vi "CMI LiB Bias Open.vi"(8 "error in":errorcluster, 10 "reset (false)":bool, 11 "VISA in":refnum<visa-resource-name>) -> (0 "error out":errorcluster, 2 "idn string":string, 3 "VISA out":refnum<visa-resource-name>)   [LabVIEW 2020]
uses:
  <vilib>/Utility/error.llb/Error Cluster From Error Code.vi
  <vilib>/ErrorRing/Error Ring.xnode
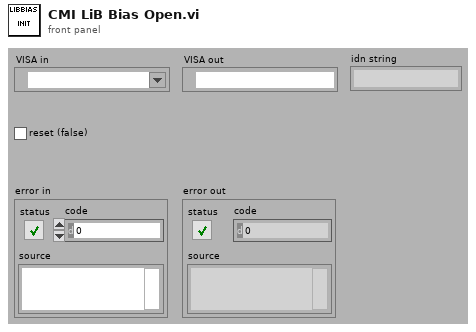
[diagram p1: front panel]
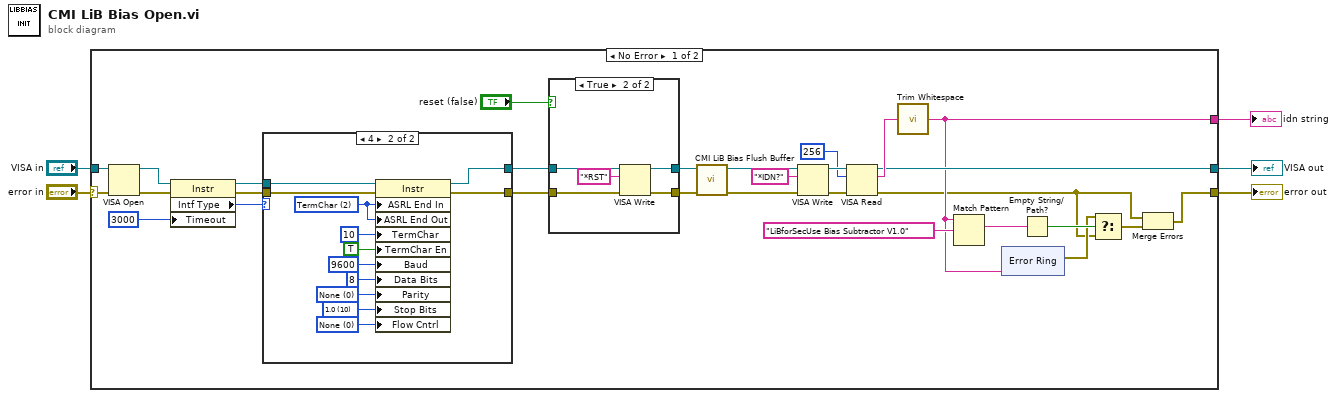
[diagram p0: block diagram]
diagram:
  n1 = case shown="No Error" "error in" {
    selector: "error in" -> [w10 w64]
    tunnel: "VISA in" -> [w34 w63]
    tunnel: [w19 w63] -> w4
    tunnel: [w17 w64] -> w3
    tunnel: [w15 _] -> w2
    frame No Error {
      n2 = VISA Open(error in (no error)=w10, VISA resource name=w34) -> (VISA resource name=w32:refnum<visa-resource-name>, error out=w33:errorcluster)  [unwired: 3 in]
      n3 = property class="Instr"(reference=w32, error in=w33, "Timeout"=u32 3000 ("General Settings:Timeout Value")) -> (reference out=w29:refnum<visa-resource-name>, error out=w30:errorcluster, "Intf Type"=w31:u16)
      n4 = case shown="4" w31 {
        tunnel: w30 -> [w50 w62]
        tunnel: w29 -> [w49 w53]
        tunnel: [w50 w52] -> w27
        tunnel: [w49 w51] -> w26
        frame Default {
        }
        frame 4 {
          w54 = u16 0 items=["None", "XON/XOFF", "RTS/CTS", "XON/XOFF & RTS/CTS", "DTR/DSR", "XON/XOFF & DTR/DSR"] ("Serial Settings:Flow Control")
          w55 = u16 10 items=["1.0"=10, "1.5"=15, "2.0"=20] ("Serial Settings:Stop Bits")
          w56 = u16 0 items=["None", "Odd", "Even", "Mark", "Space"] ("Serial Settings:Parity")
          w61 = u16 2 items=["None", "Last Bit", "TermChar"] ("Serial Settings:End Mode for Reads")
          n5 = property class="Instr"(reference=w53, error in=w62, "ASRL End In"=w61, "ASRL End Out"=w61, "TermChar"=u8 10 ("Message Based Settings:Termination Character"), "TermChar En"=TRUE ("Message Based Settings:Termination Character Enable"), "Baud"=u32 9600 ("Serial Settings:Baud Rate"), "Data Bits"=u16 8 ("Serial Settings:Data Bits"), "Parity"=w56, "Stop Bits"=w55, "Flow Cntrl"=w54) -> (reference out=w51:refnum<visa-resource-name>, error out=w52:errorcluster)
        }
      }
      n6 = case shown="True" "reset (false)" {
        tunnel: w27 -> [w42 w48]
        tunnel: w26 -> [w43 w47]
        tunnel: [w42 w45] -> w9
        tunnel: [w43 w44] -> w7
        frame False {
        }
        frame True {
          n7 = VISA Write(VISA resource name=w47, write buffer="*RST", error in (no error)=w48) -> (VISA resource name out=w44:refnum<visa-resource-name>, error out=w45:errorcluster)  [unwired: 1 out]
        }
      }
      n8 = call "CMI LiB Bias Flush Buffer.vi"("error in"=w9, "VISA in"=w7) -> ("error out"=w8:errorcluster, "VISA out"=w6:refnum<visa-resource-name>)  [unwired: 8 in]
      n9 = VISA Write(VISA resource name=w6, write buffer="*IDN?", error in (no error)=w8) -> (VISA resource name out=w22:refnum<visa-resource-name>, error out=w23:errorcluster)  [unwired: 1 out]
      n10 = VISA Read(VISA resource name=w22, byte count=u32 256, error in (no error)=w23) -> (VISA resource name out=w19:refnum<visa-resource-name>, read buffer=w20:string, error out=w11:errorcluster)  [unwired: 1 out]
      n11 = call <vilib>:"Trim Whitespace.vi"("string"=w20) -> ("trimmed string"=w15:string)  [unwired: 1 in]
      n12 = Match Pattern(string=w15, regular expression="LiBforSecUse Bias Subtractor V1.0") -> (match substring=w14:string)  [unwired: 1 in, 3 out]
      n13 = xnode "Error Ring"("parameter 0"=w15) -> ("error out"=w12:errorcluster)
      n14 = Empty String/Path?(string/path=w14) -> (empty?=w13:bool)
      n15 = Select(t=w12, s=w13, f=w11) -> (s? t:f=w16:errorcluster)
      n16 = Merge Errors(w11, w16) -> (w17:errorcluster)
    }
    frame Error {
    }
  }
  "error out" <- w3
  "VISA out" <- w4
  "idn string" <- w2
